vi "DSF.Engine.Memory.Cache.Framework.Create.vi"(7 "Plugin Cache type":refnum<class "DSF.Engine.Memory.Cache.Plugin.lvclass">, 8 "error in (no error)":errorcluster, 10 "Framework Configuration in":refnum<class "DSF.Shared.Configuration.Framework.lvclass">, 11 "Framework Cache type":refnum<class "DSF.Engine.Memory.Cache.Framework.lvclass">) -> (0 "error out":errorcluster, 3 "Framework Cache":refnum<class "DSF.Engine.Memory.Cache.Framework.lvclass">)   [LabVIEW 2016, in "DSF.Engine.lvlib" / "DSF.Engine.Memory.Cache.Framework.lvclass"]
uses:
  DSF.Engine.Memory.Cache.Framework.lvclass
  DSF.Engine.Memory.Cache.Plugin.lvclass
  Shared/Classes/Framework/DSF.Shared.Configuration.Framework.lvclass
  Shared/Classes/Framework/DSF.Shared.Configuration.Framework.lvclass/DSF.Shared.Configuration.Framework.ctl
  DSF.Engine.Memory.Cache.Framework.lvclass/DSF.Engine.Memory.Cache.Framework.ctl
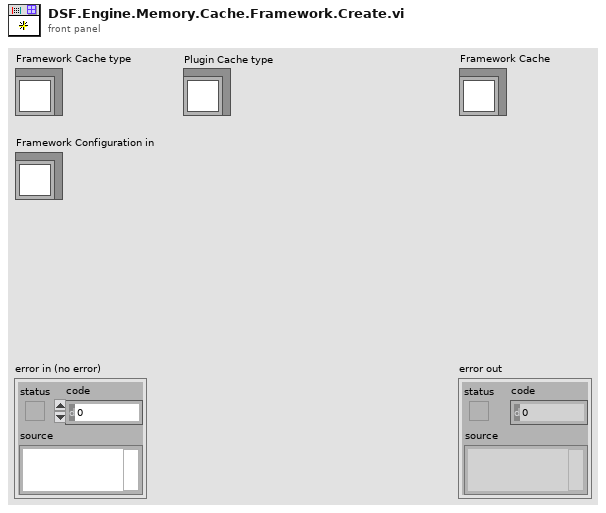
[diagram p1: front panel]
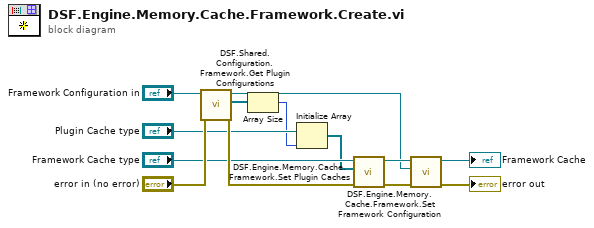
[diagram p0: block diagram]
diagram:
  n1 = call "DSF.Shared.Configuration.Framework.Get Plugin Configurations.vi"("error in (no error)"="error in (no error)", "Framework Configuration in"="Framework Configuration in") -> ("error out"=w13:errorcluster, "Plugin Configurations"=w10:refnum<class "DSF.Shared.Configuration.Plugin.lvclass">[], "Framework Configuration out"=w1:refnum<class "DSF.Shared.Configuration.Framework.lvclass">)  [unwired: 7 in]
  n2 = Array Size(array=w10) -> (size(s)=w9:i32)
  n3 = Initialize Array("Plugin Cache type", w9) -> (w2:refnum<class "DSF.Engine.Memory.Cache.Plugin.lvclass">[])
  n4 = call "DSF.Engine.Memory.Cache.Framework.Set Plugin Caches.vi"("error in (no error)"=w13, "Plugin Caches"=w2, "Framework Cache in"="Framework Cache type") -> ("error out"=w4:errorcluster, "Framework Cache out"=w7:refnum<class "DSF.Engine.Memory.Cache.Framework.lvclass">)  [unwired: 7 in]
  n5 = call "DSF.Engine.Memory.Cache.Framework.Set Framework Configuration.vi"("error in (no error)"=w4, "Framework Configuration"=w1, "Framework Cache in"=w7) -> ("error out"=→"error out":errorcluster, "Framework Cache out"=→"Framework Cache":refnum<class "DSF.Engine.Memory.Cache.Framework.lvclass">)  [unwired: 7 in]
